vi "Acquire AI.vi"(8 "error in (no error)":errorcluster, 11 "PXIe 6363 in":refnum<class "PXIe 6363.lvclass">) -> (0 "error out":errorcluster, 1 "data":waveform(dbl)[](array[waveform]), 2 "Waveform Graph":dbl[][](graph), 3 "PXIe 6363 out":refnum<class "PXIe 6363.lvclass">)   [LabVIEW 2021, in "DAQ Hardware.lvlib" / "PXIe 6363.lvclass"]
uses:
  PXIe 6363.lvclass
  PXIe 6363.lvclass/PXIe 6363.ctl
  <vilib>/DAQmx/read.llb/DAQmx Read (Analog 1D Wfm NChan NSamp).vi
  <vilib>/DAQmx/miscellaneous.llb/DAQmx Fill In Error Info.vi
  DAQ Hardware.lvlib
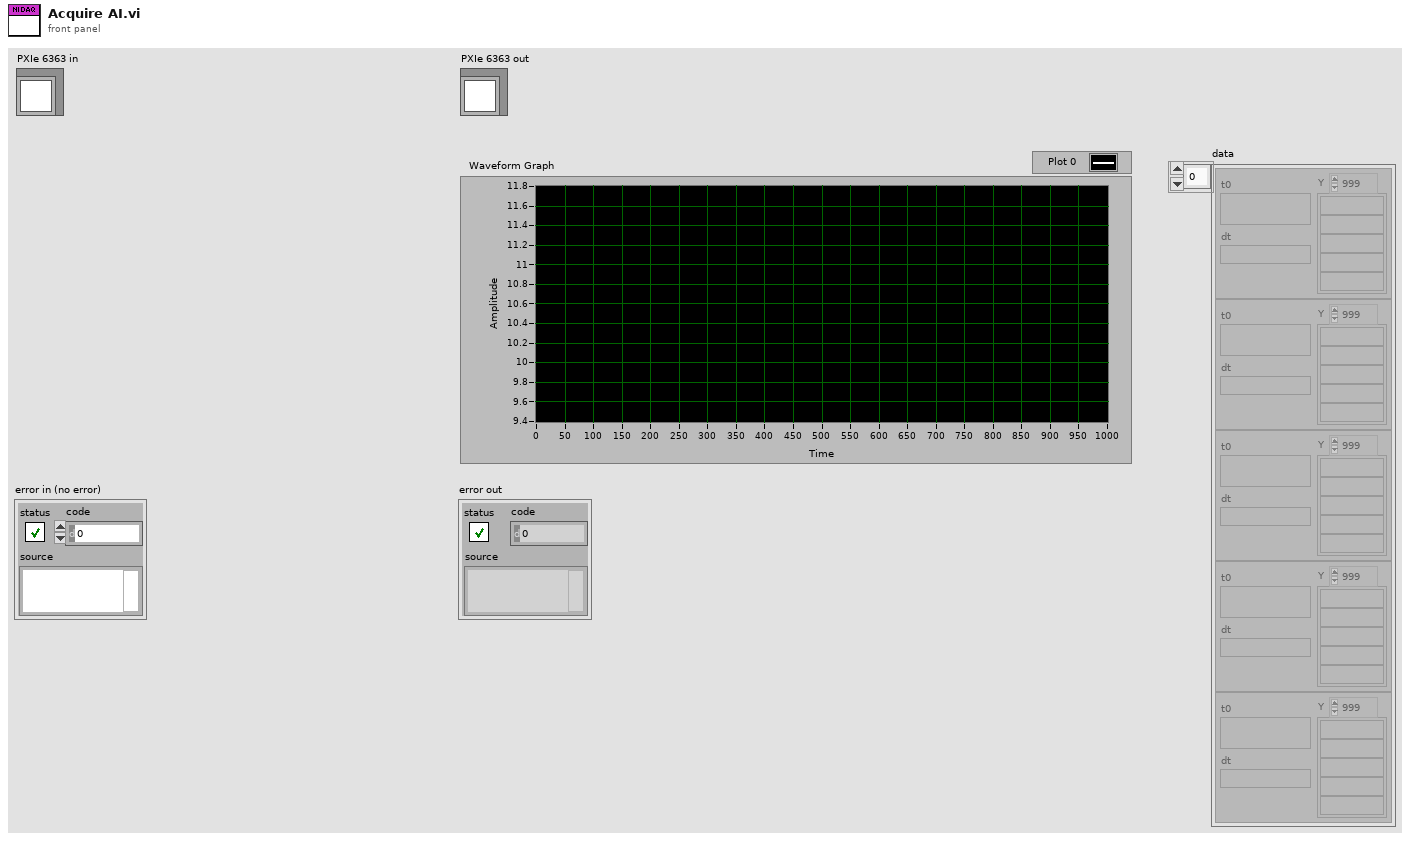
[diagram p1: front panel]
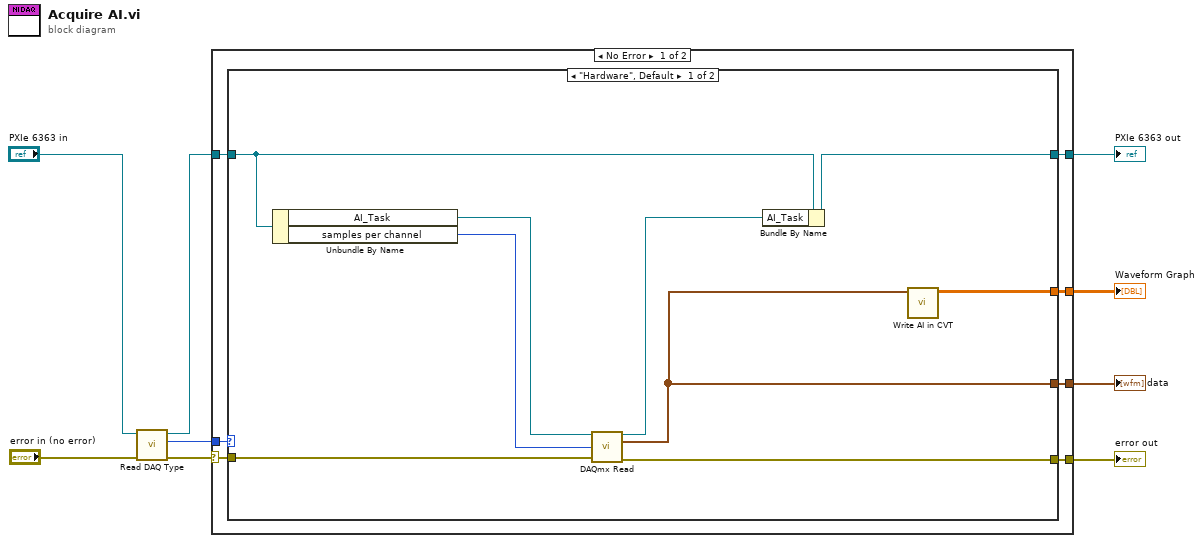
[diagram p0: block diagram]
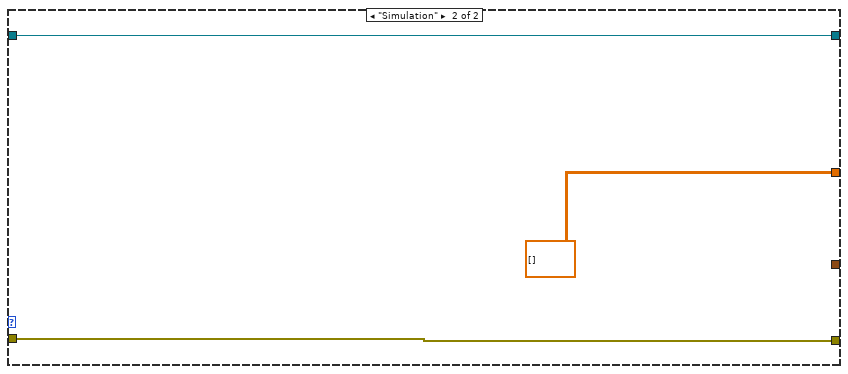
[diagram p2: hidden frame]
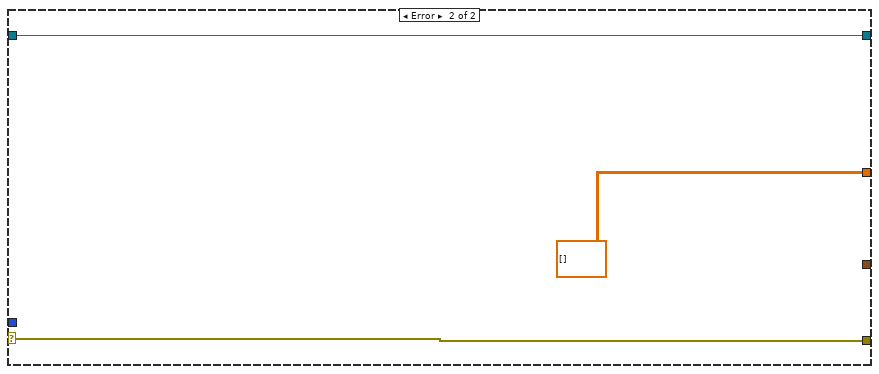
[diagram p3: hidden frame]
diagram:
  n1 = call-dynamic "Read DAQ Type.vi"("error in (no error)"="error in (no error)", "PXIe 6363 in"="PXIe 6363 in") -> ("error out"=w8:errorcluster, "DAQ Type"=w7:enum16{"Hardware", "Simulation"}, "PXIe 6363 out"=w1:refnum<class "PXIe 6363.lvclass">)  [unwired: 7 in]
  n2 = case shown="No Error" w8 {
    selector: w8 -> [w15 w30]
    tunnel: w7 -> [w16 _]
    tunnel: w1 -> [w14 w31]
    tunnel: [w13 w31] -> w5
    tunnel: [w12 w30] -> w4
    tunnel: [w11 dbl[][] [] ("data")] -> w3
    tunnel: [w10 _] -> w2
    frame No Error {
      n3 = case shown="\"Hardware\", Default" w16 {
        tunnel: w15 -> [w23 w27]
        tunnel: w14 -> [w25 w28]
        tunnel: [w24 w28] -> w13
        tunnel: [w21 w27] -> w12
        tunnel: [w22 dbl[][] [] ("data")] -> w11
        tunnel: [w20 _] -> w10
        frame "Hardware", Default {
          n4 = Unbundle By Name(w25) -> ("AI_Task"=w19:refnum<k21>, "samples per channel"=w17:i32)
          n5 = call-poly <vilib>:"DAQmx Read.vi"("task/channels in"=w19, "number of samples per channel"=w17, "error in"=w23) -> ("task out"=w18:refnum<k21>, "data"=w20:waveform(dbl)[], "error out"=w21:errorcluster)  [unwired: 10 in]
          n6 = Bundle By Name(cluster=w25, "AI_Task"=w18) -> (w24:refnum<class "PXIe 6363.lvclass">)
          n7 = call "Write AI in CVT.vi"("Data In"=w20) -> ("Data Out"=w22:dbl[][])  [unwired: 10 in]
        }
        frame "Simulation" {
        }
      }
    }
    frame Error {
    }
  }
  "error out" <- w4
  "PXIe 6363 out" <- w5
  "Waveform Graph" <- w3
  "data" <- w2
